vi "StopExperiment.vi"(10 "Stop Values":T1, 11 "Experiment In":T2={"File Path"=path "", "Operator"="Operator", "Project"="Project Description", "Target Dose (dpa)"=nan, "Sample"={"Name"="", "Description"="", "Molar Mass (g/mol)"=nan, "Density (g/cm^3)"=nan, "Irradiation Area (cm^2)"=nan, "SRIM Damage Peak (disp * ions/cm)"=nan}, "Beam Line"={"Type"=enum."Ion Beam Analysis", "Ion"=enum."H", "Charge State"=0, "Total Source Ion Energy (kV)"=nan}, "Runs"=[]} {"Beam Line"."Charge State" min=1}) -> (3 "Experiment Out":T2={"File Path"=path "", "Operator"="Operator", "Project"="Project Description", "Target Dose (dpa)"=nan, "Sample"={"Name"="", "Description"="", "Molar Mass (g/mol)"=nan, "Density (g/cm^3)"=nan, "Irradiation Area (cm^2)"=nan, "SRIM Damage Peak (disp * ions/cm)"=nan}, "Beam Line"={"Type"=enum."Ion Beam Analysis", "Ion"=enum."H", "Charge State"=0, "Total Source Ion Energy (kV)"=nan}, "Runs"=[]} {"Beam Line"."Charge State" min=1})   [LabVIEW 2012]
uses:
  Experiment.ctl
  Sample.ctl
  BeamLine.ctl
  BeamLineType.ctl
  BeamLineIon.ctl
  ExperimentRun.ctl
  ExperimentRunTiming.ctl
  ExperimentRunDose.ctl
  ExperimentRunFluence.ctl
  ExperimentRunTotalCharge.ctl
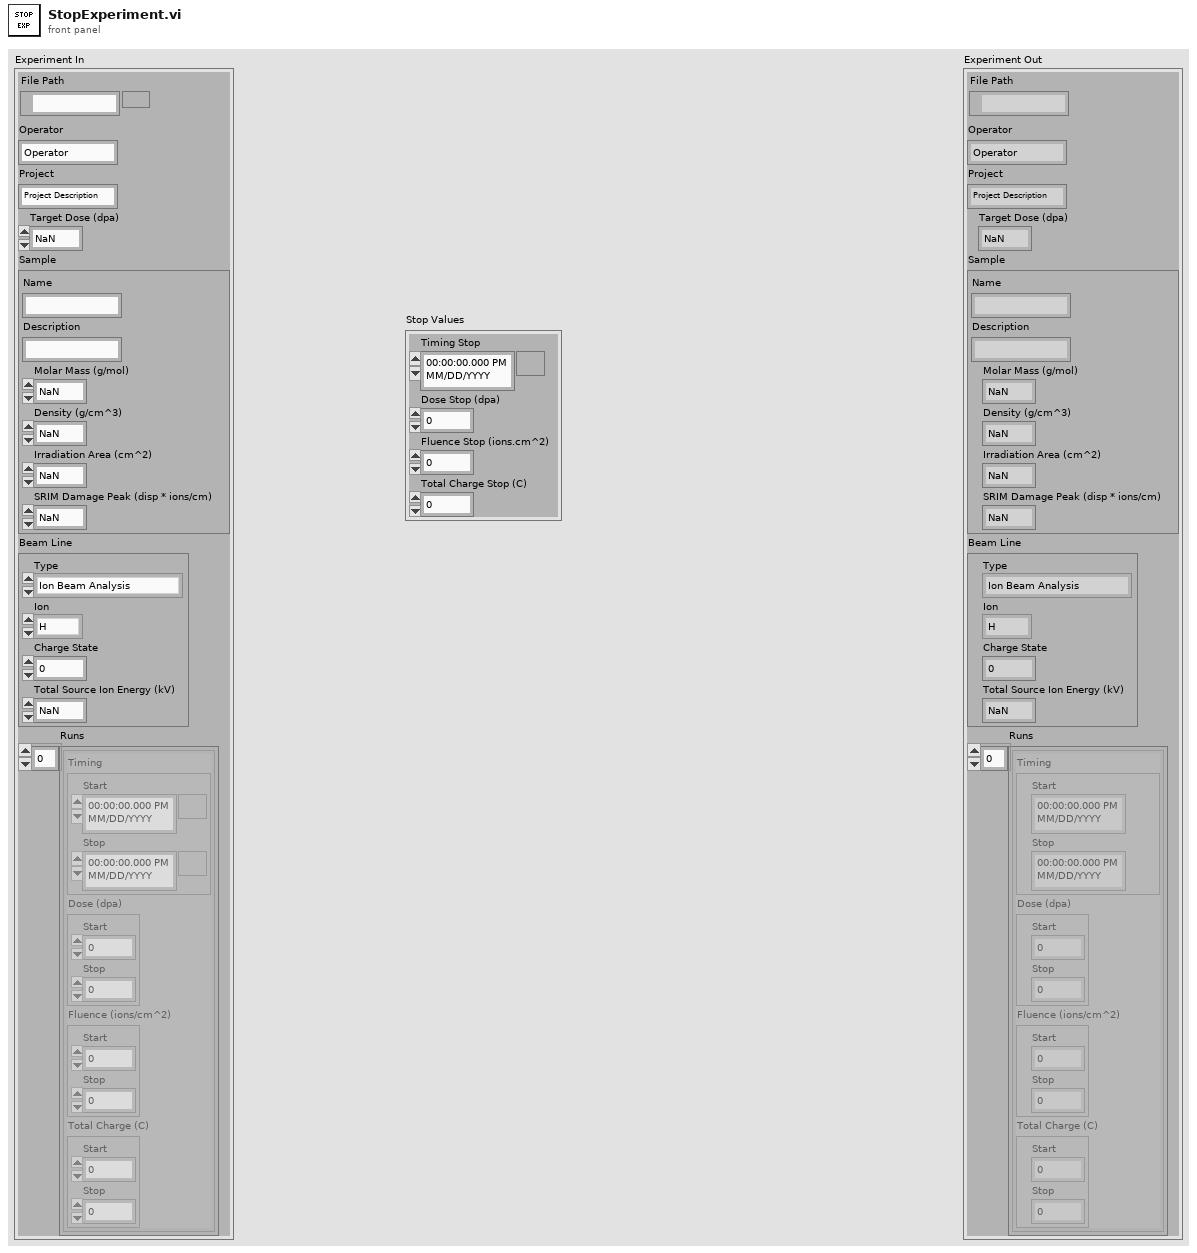
[diagram p1: front panel]
types:
  T1 = cluster{"Timing Stop":timestamp, "Dose Stop (dpa)":dbl, "Fluence Stop (ions.cm^2)":dbl, "Total Charge Stop (C)":dbl}
  T2 = typedef "Experiment.ctl" = cluster{"File Path":path, "Operator":string, "Project":string, "Target Dose (dpa)":dbl, "Sample":T3, "Beam Line":T4, "Runs":T7[]}
  T3 = typedef "Sample.ctl" = cluster{"Name":string, "Description":string, "Molar Mass (g/mol)":dbl, "Density (g/cm^3)":dbl, "Irradiation Area (cm^2)":dbl, "SRIM Damage Peak (disp * ions/cm)":dbl}
  T4 = typedef "BeamLine.ctl" = cluster{"Type":T5, "Ion":T6, "Charge State":u8, "Total Source Ion Energy (kV)":dbl}
  T5 = typedef "BeamLineType.ctl" = enum16{"Ion Beam Analysis", "Auxiliary", "Radiation Damage"}
  T6 = typedef "BeamLineIon.ctl" = enum16{"H", "He", "C", "Fe", "Ni", "Pt", "Si", "Ag", "Au"}
  T7 = typedef "ExperimentRun.ctl" = cluster{"Timing":T8, "Dose (dpa)":T9, "Fluence (ions/cm^2)":T10, "Total Charge (C)":T11}
  T8 = typedef "ExperimentRunTiming.ctl" = cluster{"Start":timestamp, "Stop":timestamp}
  T9 = typedef "ExperimentRunDose.ctl" = cluster{"Start":dbl, "Stop":dbl}
  T10 = typedef "ExperimentRunFluence.ctl" = cluster{"Start":dbl, "Stop":dbl}
  T11 = typedef "ExperimentRunTotalCharge.ctl" = cluster{"Start":dbl, "Stop":dbl}
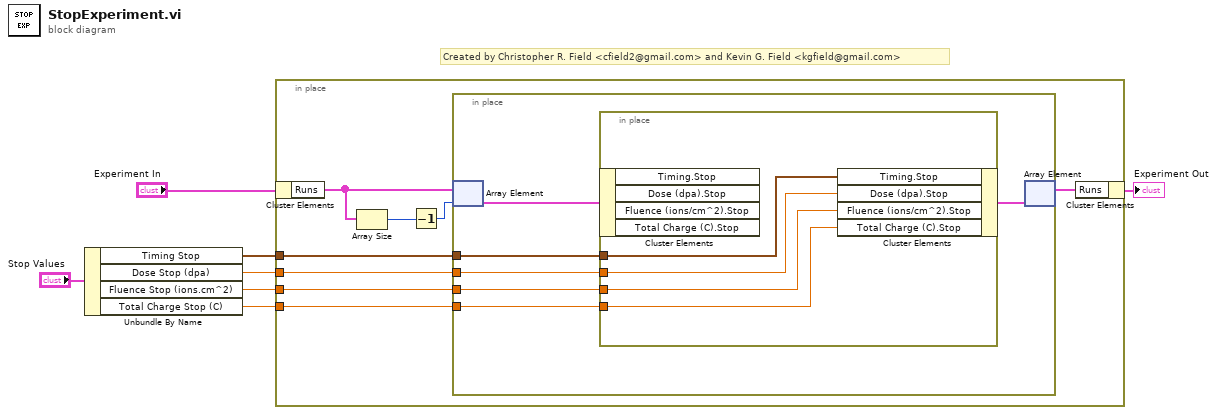
[diagram p0: block diagram]
diagram:
  # "Created by Christopher R. Field <cfield2@gmail.com> and Kevin G. Field <kgfield@gmail.com>"
  n1 = Unbundle By Name("Stop Values") -> ("Timing Stop"=w4:timestamp, "Dose Stop (dpa)"=w3:dbl, "Fluence Stop (ions.cm^2)"=w2:dbl, "Total Charge Stop (C)"=w1:dbl)
  n2 = in-place {
    in-place-border: w4 -> [w11]
    in-place-border: w3 -> [w10]
    in-place-border: w2 -> [w9]
    in-place-border: w1 -> [w8]
    n3 = in-place-cluster #1("Experiment In") -> ("Runs"=w13:T7[])
    n4 = Array Size(array=w13) -> (size(s)=w15:i32)
    n5 = Decrement(x=w15) -> (x-1=w14:i32)
    n6 = in-place {
      in-place-border: w11 -> [w19]
      in-place-border: w10 -> [w18]
      in-place-border: w9 -> [w17]
      in-place-border: w8 -> [w16]
      n7 = in-place-array #2(w13, w14) -> (w21:T7)
      n8 = in-place {
        in-place-border: w19 -> [w25]
        in-place-border: w18 -> [w24]
        in-place-border: w17 -> [w23]
        in-place-border: w16 -> [w22]
        n9 = in-place-cluster #3(w21) -> ()  [unwired: 4 out]
        n10 = in-place-cluster #3("Timing.Stop"=w25, "Dose (dpa).Stop"=w24, "Fluence (ions/cm^2).Stop"=w23, "Total Charge (C).Stop"=w22) -> (w20:T7)
      }
      n11 = in-place-array #2(w20) -> (w12:T7[])  [unwired: 1 out]
    }
    n12 = in-place-cluster #1("Runs"=w12) -> (→"Experiment Out":T2)
  }
